vi "Example - File.vi"   [LabVIEW 2020, in "Global_logger.lvlib"]
uses:
  Global_logger.lvlib
  File Options.ctl
  Levels.ctl
  New TSV Logger.vi
types:
  T1 = typedef "Global_logger.lvlib/Levels.ctl" = enum16{"ALL", "TRACE", "DEBUG", "INFO", "WARN", "ERROR", "FATAL", "OFF"}
  T2 = typedef "Global_logger.lvlib/File Options.ctl" = cluster{"filesize (bytes)":u32, "logs max age (days) ":i32, "Filename":string, "Root path":path}
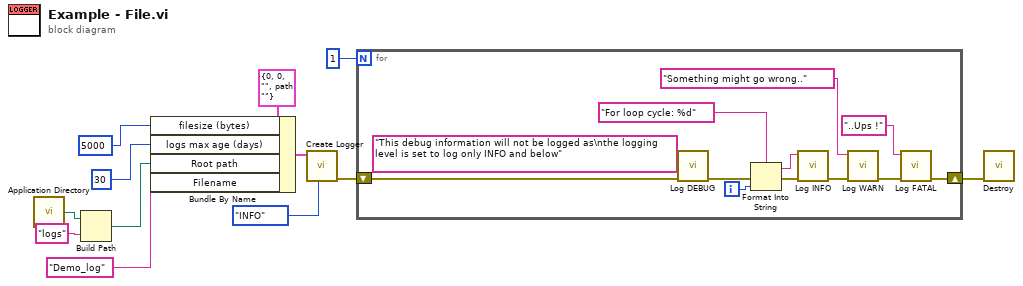
[diagram p0: block diagram]
diagram:
  n1 = call <vilib>:"Application Directory.vi"() -> ("Application Directory"=w12:path)
  n2 = Build Path(base path=w12, name or relative path="logs") -> (appended path=w3:path)
  n3 = Bundle By Name(cluster=T2 {"filesize (bytes)"=0, "logs max age (days) "=0, "Filename"="", "Root path"=path ""} ("File Options"), "filesize (bytes)"=u32 5000, "logs max age (days)"=30, "Root path"=w3, "Filename"="Demo_log") -> (w6:T2)
  n4 = call-poly "Create Logger.vi"("Level"=Levels."INFO", "File Options"=w6) -> ("error out"=w8:errorcluster)  [unwired: 9 in]
  n5 = for {
    N: 1 -> [_]
    shift-right: [w21] -> w10
    shift-left: w8 -> [w24]
    i -> [w17]
    n6 = call "Log DEBUG.vi"("error in (no error)"=w24, "Message"="This debug information will not be logged as\nthe logging level is set to log only INFO and below") -> ("error out"=w23:errorcluster)  [unwired: 9 in]
    n7 = Format Into String(format string="For loop cycle: %d", error in=w23, w17) -> (resulting string=w15:string, error out=w18:errorcluster)  [unwired: 1 in]
    n8 = call "Log INFO.vi"("error in (no error)"=w18, "Message"=w15) -> ("error out"=w22:errorcluster)  [unwired: 9 in]
    n9 = call "Log WARN.vi"("error in (no error)"=w22, "Message"="Something might go wrong.." ("format string")) -> ("error out"=w14:errorcluster)  [unwired: 9 in]
    n10 = call "Log FATAL.vi"("error in (no error)"=w14, "Message"="..Ups !") -> ("error out"=w21:errorcluster)  [unwired: 9 in]
  }
  n11 = call "Destroy.vi"("error in (no error)"=w10) -> ()  [unwired: 10 in, 1 out]
